vi "Controller Fast Command Receive and Split.vi"(0 "Fast Command FIFO":refnum<k33>, 5 "Fast Command Enabled":bool, 11 "error in (no error)":errorcluster) -> (4 "FC Data":sgl[](array[numeric]), 6 "FC BPM Mode":u16, 8 "FC PS Mode":u16, 10 "FC Marker":u32, 15 "error out":errorcluster)   [LabVIEW 2011, in "Controller VIs.lvlib"]
uses:
  Controller VIs.lvlib
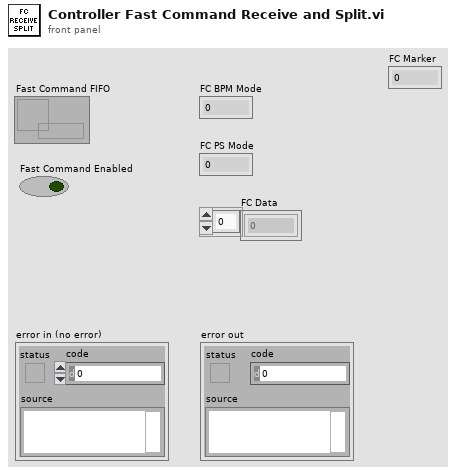
[diagram p1: front panel]
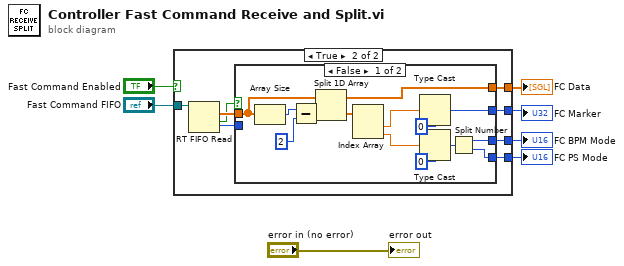
[diagram p0: block diagram]
diagram:
  n1 = case shown="True" "Fast Command Enabled" {
    tunnel: "Fast Command FIFO" -> [_ w15]
    tunnel: [_ w14] -> w7
    tunnel: [_ w13] -> w4
    tunnel: [_ w12] -> w6
    tunnel: [_ w8] -> w1
    frame False {
    }
    frame True {
      n2 = RT FIFO Read(0:w15) -> (7:w10:u32, 9:w11:sgl[], 10:w9:bool)  [unwired: 3 in, 2 out]
      n3 = case shown="False" w9 {
        tunnel: [w29 _] -> w14
        tunnel: [w26 _] -> w13
        tunnel: [w25 _] -> w12
        tunnel: w11 -> [w24 _]
        tunnel: w10 -> [_ _]
        tunnel: [w20 _] -> w8
        frame False {
          n4 = Array Size(array=w24) -> (size(s)=w17:i32)
          n5 = Subtract(x=w17, y=2) -> (x-y=w28:i32)
          n6 = Split 1D Array(array=w24, index=w28) -> (first subarray=w29:sgl[], second subarray=w23:sgl[])
          n7 = Index Array(array=w23) -> (element #1=w19:sgl, element #2=w18:sgl)  [unwired: 2 in]
          n8 = Type Cast(type=u32 0, x=w19) -> (*(type *) &x=w20:u32)
          n9 = Type Cast(type=u32 0, x=w18) -> (*(type *) &x=w21:u32)
          n10 = Split Number(x=w21) -> (hi(x)=w26:u16, lo(x)=w25:u16)
        }
        frame True {
        }
      }
    }
  }
  "FC Data" <- w7
  "FC PS Mode" <- w6
  "FC BPM Mode" <- w4
  "FC Marker" <- w1
  "error out" <- "error in (no error)"
